vi "example2-ParamClusterControl.vi"() -> ()   [LabVIEW 2021]
panel:
  in  "String":string
  in  "Cluster 2":cluster{"Numeric":dbl}
  in  "Cluster":cluster{"Numeric":dbl}
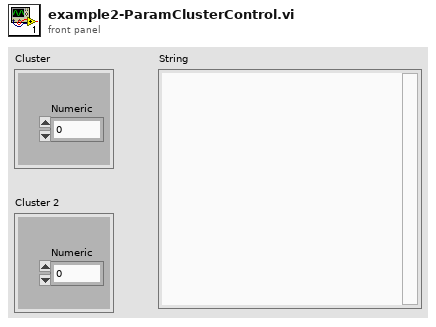
[diagram p1: front panel]
types:
  T1 = cluster{"Operation":enum16{"read", "write"}, "Data":string, "Queue":refnum<queue>}
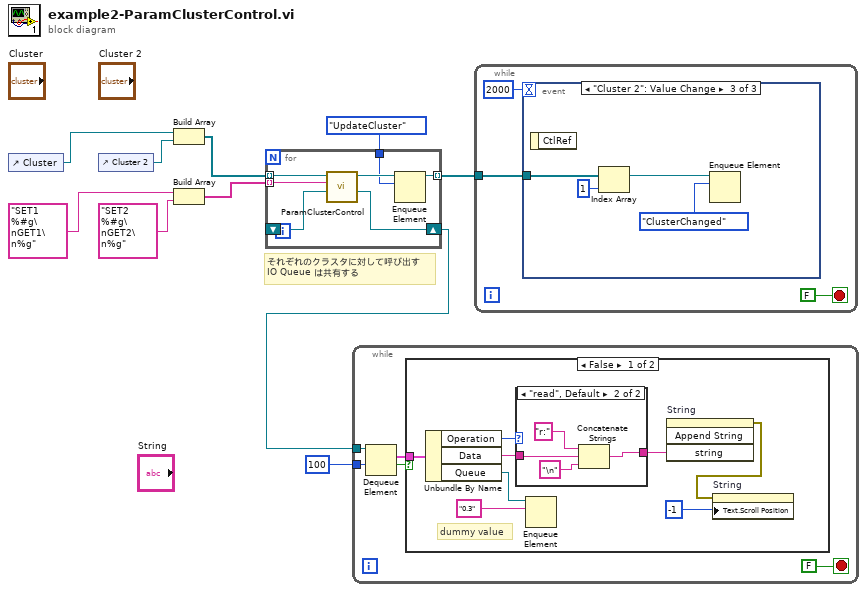
[diagram p0: block diagram]
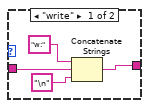
[diagram p2: hidden frame]
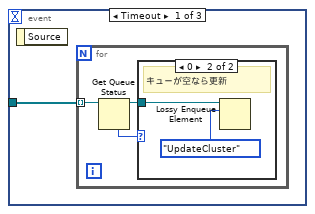
[diagram p4: hidden frame]
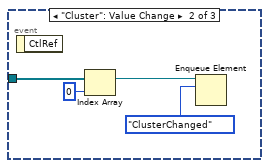
[diagram p6: hidden frame]
diagram:
  # "それぞれのクラスタに対して呼び出す\nIO Queue は共有する"
  n1 = control-ref of="Cluster"() -> (w8:refnum<vi>)
  n2 = control-ref of="Cluster 2"() -> (w7:refnum<vi>)
  n3 = Build Array(w8, w7) -> (w4:refnum<vi>[])
  n4 = Build Array("SET1 %#g\nGET1\n%g", "SET2 %#g\nGET2\n%g") -> (w3:string[])
  n5 = for {
    tunnel: enum16{"UpdateCluster", "ClusterChanged"}."UpdateCluster" ("element") -> [w15]
    tunnel: [w14] -> w9 mode=indexing
    tunnel: w4 -> [w13] mode=indexing
    tunnel: w3 -> [w12] mode=indexing
    shift-right: [w11] -> w1
    shift-left: _ -> [w17]
    n6 = call "ParamClusterControl.vi"("IO queue in"=w17, "SetGetCommands"=w12, "Cluster ref"=w13) -> ("IO queue out"=w11:refnum<queue>, "Command queue"=w16:refnum<queue>)  [unwired: 7 in]
    n7 = Enqueue Element(queue=w16, element=w15) -> (queue out=w14:refnum<queue>)  [unwired: 2 in, 2 out]
  }
  n8 = while {
    tunnel: 100 ("timeout in ms (-1)") -> [w22]
    tunnel: w1 -> [w21]
    stop <- FALSE stop-if-true
    n9 = Dequeue Element(queue=w21, timeout in ms (-1)=w22) -> (element=w18:T1, timed out?=w19:bool)  [unwired: 1 in, 2 out]
    n10 = case shown="False" w19 {
      tunnel: w18 -> [w30 _]
      frame False {
        # "dummy value"
        n11 = Unbundle By Name(w30) -> ("Operation"=w29:enum16{"read", "write"}, "Data"=w28:string, "Queue"=w24:refnum<queue>)
        n12 = case shown="\"read\", Default" w29 {
          tunnel: w28 -> [w33 w37]
          tunnel: [w32 w36] -> w27
          frame "write" {
            n13 = Concatenate Strings("w:", w33, "\n" ("string")) -> (w32:string)
          }
          frame "read", Default {
            n14 = Concatenate Strings("r:", w37, "\n" ("string")) -> (w36:string)
          }
        }
        n15 = Enqueue Element(queue=w24, element="0.3") -> ()  [unwired: 2 in, 3 out]
        n16 = invoke on="String" class="Str" method="Append String"("string"=w27) -> (error out=w26:errorcluster)  [unwired: 3 in, 3 out]
        n17 = property on="String" class="Str"(error in=w26, "Text.Scroll Position"=-1) -> ()  [unwired: 1 in, 2 out]
      }
      frame True {
      }
    }
  }
  n18 = while {
    tunnel: w9 -> [w39]
    stop <- FALSE stop-if-true
    n19 = event shown="[2] \"Cluster 2\": Value Change" {
      selector: _ -> [_ _ _]
      dyn-events: _ -> [_ _ _]
      timeout: 2000 -> [_ _ _]
      tunnel: w39 -> [w42 w51 w55]
      event Timeout {
        n20 = event-data() -> ()  [unwired: 1 in, 1 out]
        n21 = for {
          tunnel: w42 -> [w45] mode=indexing
          n22 = Get Queue Status(queue=w45) -> (queue out=w43:refnum<queue>, # elements in queue=w44:i32)  [unwired: 2 in, 6 out]
          n23 = case shown="0" w44 {
            tunnel: w43 -> [_ w47]
            frame Default {
            }
            frame 0 {
              # "キューが空なら更新"
              n24 = Lossy Enqueue Element(queue=w47, element=enum16{"UpdateCluster", "ClusterChanged"}."UpdateCluster") -> ()  [unwired: 1 in, 4 out]
            }
          }
        }
      }
      event "Cluster": Value Change {
        n25 = event-data() -> ()  [unwired: 1 in, 1 out]
        n26 = Index Array(array=w51, index=0) -> (element=w49:refnum<queue>)
        n27 = Enqueue Element(queue=w49, element=enum16{"UpdateCluster", "ClusterChanged"}."ClusterChanged") -> ()  [unwired: 2 in, 3 out]
      }
      event "Cluster 2": Value Change {
        n28 = event-data() -> ()  [unwired: 1 in, 1 out]
        n29 = Index Array(array=w55, index=1) -> (element=w53:refnum<queue>)
        n30 = Enqueue Element(queue=w53, element=enum16{"UpdateCluster", "ClusterChanged"}."ClusterChanged") -> ()  [unwired: 2 in, 3 out]
      }
    }
  }
